vi "FinalizeTurn.vi"(6 "Error":errorcluster, 7 "Actor":refnum<class "Actor.lvclass">, 11 "Actor":T1) -> (2 "Teardown":bool, 3 "Actor":T1, 4 "Error":errorcluster, 5 "Actor":refnum<class "Actor.lvclass">)   [LabVIEW 2020, in "jettl.lvlib"]
uses:
  jettl.lvlib
  Actor/Actor.lvclass
  Metadata/Metadata.lvclass
  Msg/Msg.lvclass
  Lifecycle.ctl
  Msg.ctl
  PostSetup.ctl
  PreSetup.ctl
  MsgNames.ctl
  ActorAttribs.ctl
  ChildActors.ctl
  Actor.ctl
  Origin.ctl
  MsgAttribs.ctl
  MsgExecuteType.ctl
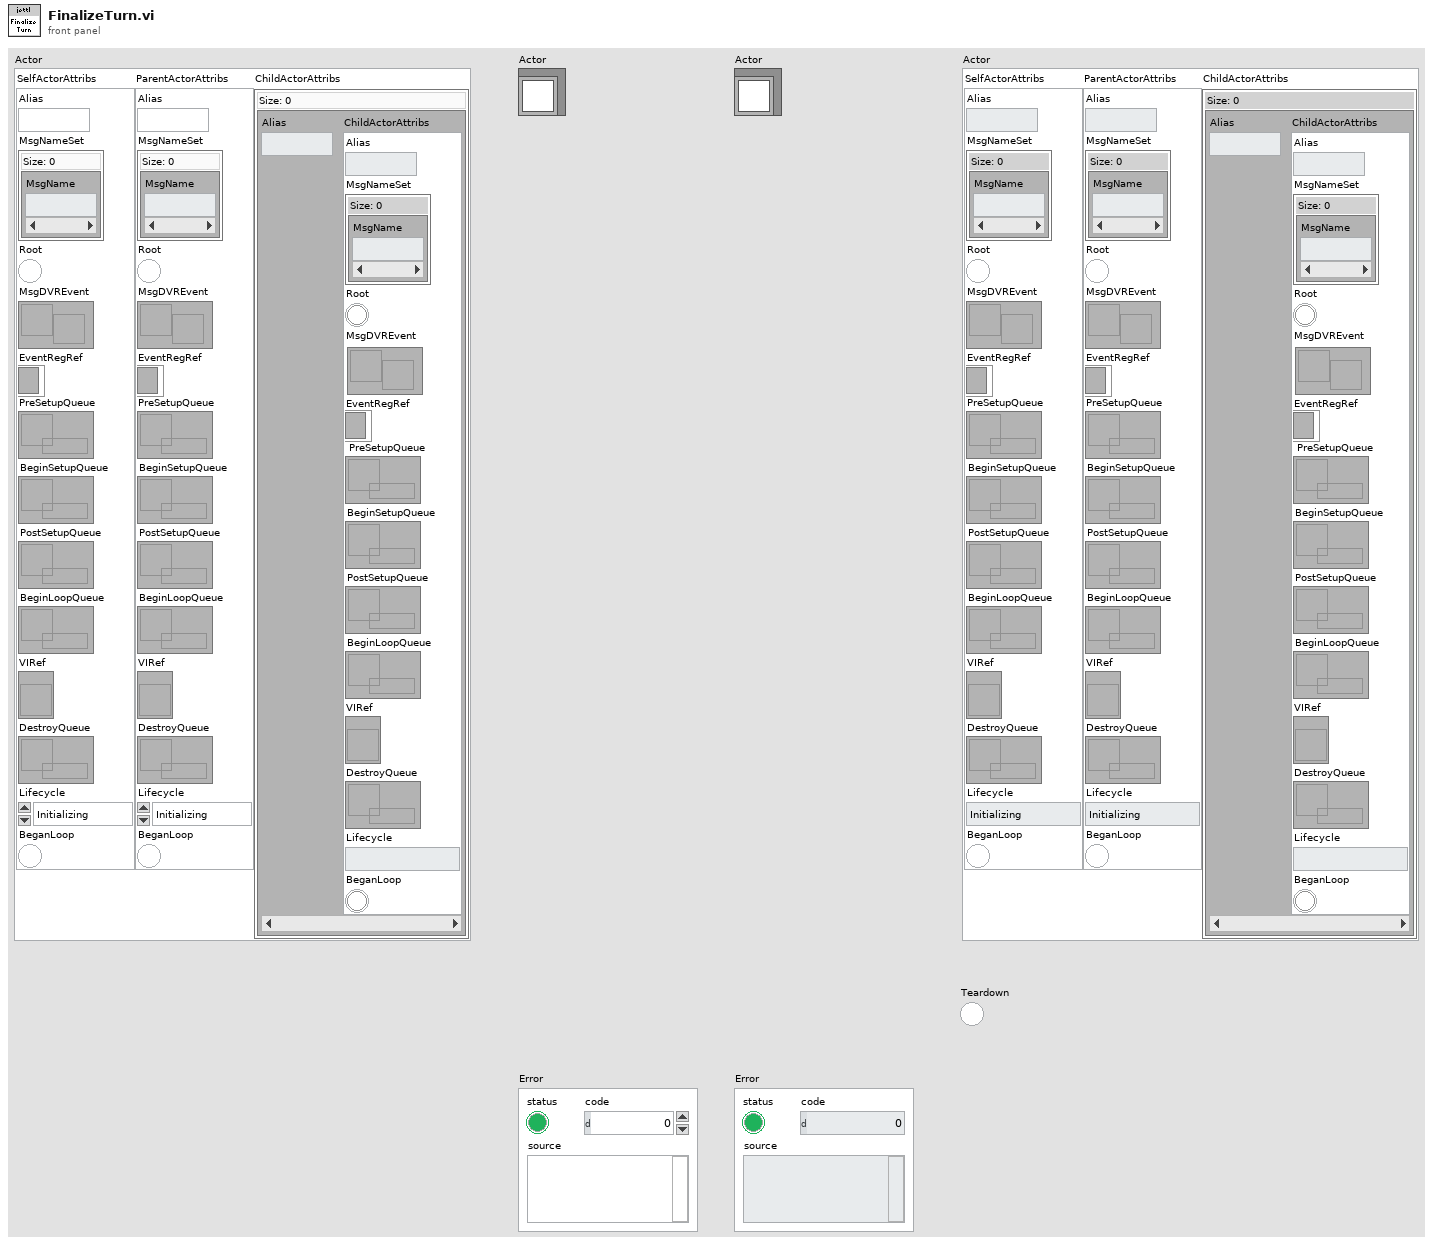
[diagram p1: front panel]
types:
  T1 = typedef "jettl.lvlib/Actor.ctl" = cluster{"SelfActorAttribs":T2, "ParentActorAttribs":T2, "ChildActorAttribs":T5}
  T2 = typedef "jettl.lvlib/ActorAttribs.ctl" = cluster{"Alias":string, "MsgNameSet":T3, "Root":bool, "MsgDVREvent":refnum<user-event>, "EventRegRef":refnum<event-registration>, "PreSetupQueue":refnum<queue>, "BeginSetupQueue":refnum<queue>, "PostSetupQueue":refnum<queue>, "BeginLoopQueue":refnum<queue>, "VIRef":refnum<vi>, "DestroyQueue":refnum<queue>, "Lifecycle":T4, "BeganLoop":bool}
  T3 = typedef "jettl.lvlib/MsgNames.ctl" = set{string}
  T4 = typedef "jettl.lvlib/Lifecycle.ctl" = enum16{"Initializing", "SettingUp", "Starting", "Running", "Stopping", "TearingDown", "Terminated"}
  T5 = typedef "jettl.lvlib/ChildActors.ctl" = map{string, T2}
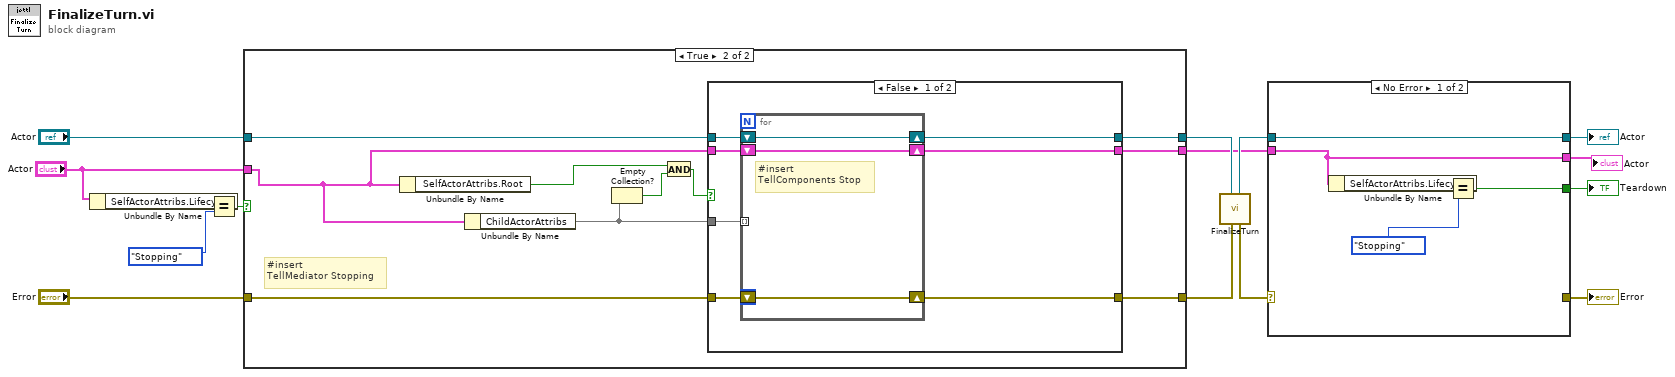
[diagram p0: block diagram]
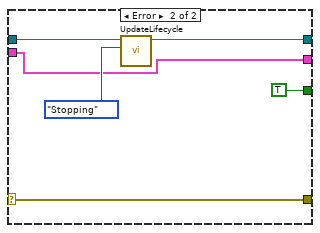
[diagram p4: hidden frame]
diagram:
  n1 = Unbundle By Name("Actor") -> ("SelfActorAttribs.Lifecycle"=w12:T4)
  n2 = Equal?(x=w12, y=Lifecycle."Stopping") -> (x = y?=w14:bool)
  n3 = case shown="True" w14 {
    tunnel: "Error" -> [w18 w27]
    tunnel: [w18 w28] -> w9
    tunnel: [w17 w25] -> w10
    tunnel: "Actor" -> [w17 w24]
    tunnel: "Actor" -> [w16 w20]
    tunnel: [w16 w19] -> w2
    frame False {
    }
    frame True {
      # "#insert\nTellMediator Stopping"
      n4 = Unbundle By Name(w20) -> ("SelfActorAttribs.Root"=w21:bool)
      n5 = Unbundle By Name(w20) -> ("ChildActorAttribs"=w26:T5)
      n6 = Empty Collection?(1:w26) -> (0:w23:bool)
      n7 = And(x=w21, y=w23) -> (x .and. y?=w22:bool)
      n8 = case shown="False" w22 {
        tunnel: w27 -> [w35 w40]
        tunnel: [w34 w40] -> w28
        tunnel: w24 -> [w33 w41]
        tunnel: [w32 w41] -> w25
        tunnel: w26 -> [w31 _]
        tunnel: w20 -> [w30 w39]
        tunnel: [w29 w39] -> w19
        frame False {
          n9 = for {
            tunnel: w31 -> [_] mode=indexing
            shift-right: [w37] -> w34
            shift-left: w35 -> [w37]
            shift-right: [w38] -> w32
            shift-left: w33 -> [w38]
            shift-right: [w36] -> w29
            shift-left: w30 -> [w36]
            # "#insert\nTellComponents Stop"
          }
        }
        frame True {
        }
      }
    }
  }
  n10 = call-dynamic "FinalizeTurn.vi"("Error"=w9, "Actor"=w10) -> ("Error"=w8:errorcluster, "Actor"=w7:refnum<class "Actor.lvclass">)  [unwired: 8 in]
  n11 = case shown="No Error" w8 {
    selector: w8 -> [_ w52]
    tunnel: [_ w52] -> w15
    tunnel: w7 -> [w45 w50]
    tunnel: [w45 w51] -> w6
    tunnel: [w44 TRUE] -> w5
    tunnel: w2 -> [w42 w47]
    tunnel: [w42 w47] -> w1
    frame No Error {
      n12 = Unbundle By Name(w42) -> ("SelfActorAttribs.Lifecycle"=w46:T4)
      n13 = Equal?(x=w46, y=Lifecycle."Stopping") -> (x = y?=w44:bool)
    }
    frame Error {
      n14 = call "UpdateLifecycle.vi"("Lifecycle"=Lifecycle."Stopping", "Actor"=w50) -> ("Actor"=w51:refnum<class "Actor.lvclass">)  [unwired: 9 in]
    }
  }
  "Actor" <- w6
  "Teardown" <- w5
  "Error" <- w15
  "Actor" <- w1
